vi "Initialise Picture Ring Array.vi"(8 "error in (no error)":errorcluster, 10 "Selection Grid":T1) -> (0 "error out":errorcluster, 1 "Valid":bool, 3 "Grassfire 2D out":refnum<class "Grassfire 2D.lvclass">)   [LabVIEW 2019, in "Grassfire 2D.lvclass"]
uses:
  Grassfire 2D.lvclass
  Shared/Selection--array.ctl
  Shared/Selection--picture ring.ctl
  Node Address--cluster.ctl
  Node Value--cluster.ctl
  Shared/Node Type--enum.ctl
  Grassfire 2D.lvclass/Grassfire 2D.ctl
  Shared/Shared.lvlib
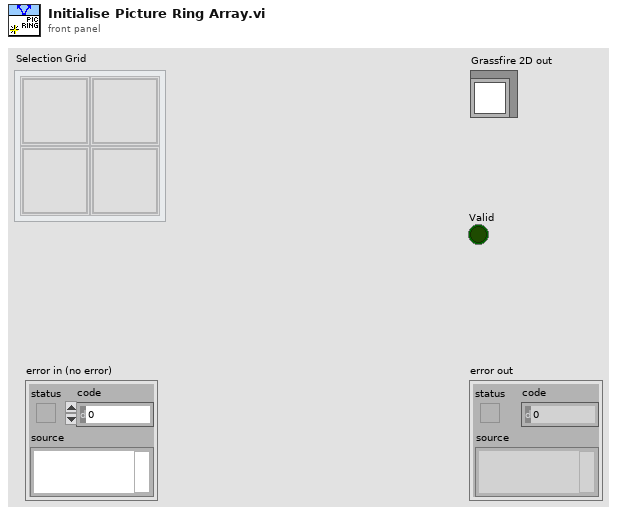
[diagram p1: front panel]
types:
  T1 = typedef "Shared.lvlib/Selection--array.ctl" = cluster{"Grid Value":T2}[][]
  T2 = typedef "Shared.lvlib/Selection--picture ring.ctl" = i64
  T3 = typedef "Grassfire 2D.lvclass/Node Address--cluster.ctl" = cluster{"Row":i32, "Column":i32}
  T4 = typedef "Grassfire 2D.lvclass/Node Value--cluster.ctl" = cluster{"Type":T5, "Distance":i32}
  T5 = typedef "Shared.lvlib/Node Type--enum.ctl" = enum16{"Empty", "Blocked", "Start", "End", "Path"}
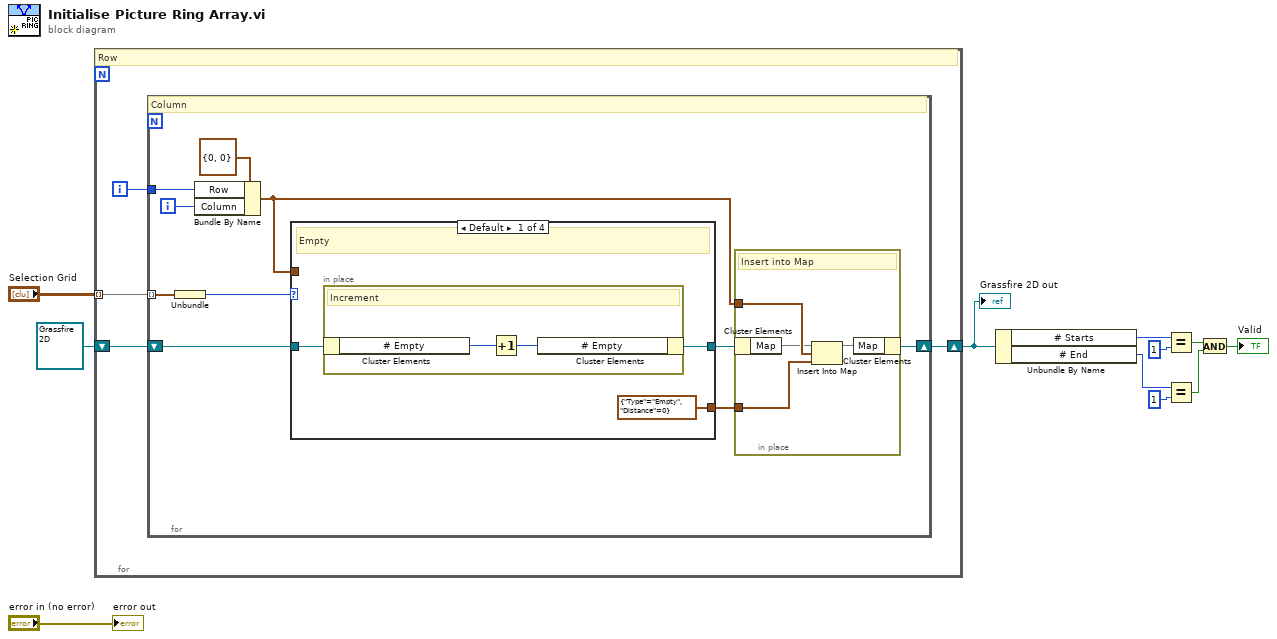
[diagram p0: block diagram]
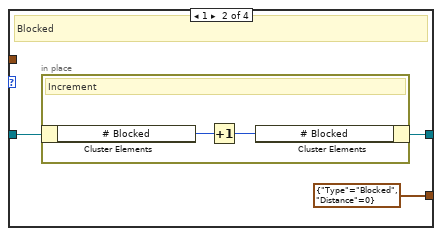
[diagram p2: hidden frame]
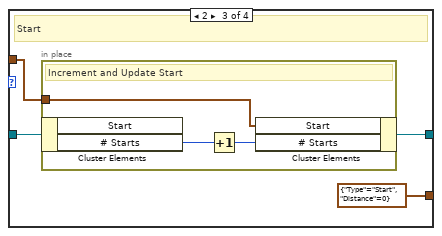
[diagram p3: hidden frame]
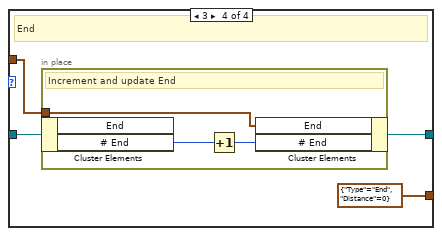
[diagram p4: hidden frame]
diagram:
  n1 = for {
    shift-right: [w13] -> w2
    shift-left: refnum<class "Grassfire 2D.lvclass"> refnum ("Grassfire 2D out") -> [w15]
    tunnel: "Selection Grid" -> [w14] mode=indexing
    i -> [w12]
    # "Row"
    n2 = for {
      shift-right: [w21] -> w13
      shift-left: w15 -> [w23]
      tunnel: w14 -> [w25] mode=indexing
      tunnel: w12 -> [w19]
      i -> [w18]
      # "Column"
      n3 = Unbundle(w25) -> ("Grid Value"=w24:T2)
      n4 = Bundle By Name(cluster=T3 {"Row"=0, "Column"=0} ("Address"), "Row"=w19, "Column"=w18) -> (w16:T3)
      n5 = case shown="Default" w24 {
        tunnel: w23 -> [w32 w37 w43 w50]
        tunnel: [w31 w36 w42 w49] -> w22
        tunnel: [T4 {"Type"=enum."Empty", "Distance"=0} ("Value") T4 {"Type"=enum."Blocked", "Distance"=0} ("Value") T4 {"Type"=enum."Start", "Distance"=0} ("Value") T4 {"Type"=enum."End", "Distance"=0} ("Value")] -> w17
        tunnel: w16 -> [_ _ w40 w48]
        frame Default {
          # "Empty"
          n6 = in-place {
            # "Increment"
            n7 = in-place-cluster #1(w32) -> ("# Empty"=w34:i32)
            n8 = Increment(x=w34) -> (x+1=w33:i32)
            n9 = in-place-cluster #1("# Empty"=w33) -> (w31:refnum<class "Grassfire 2D.lvclass">)
          }
        }
        frame 1 {
          # "Blocked"
          n10 = in-place {
            # "Increment"
            n11 = in-place-cluster #2(w37) -> ("# Blocked"=w39:i32)
            n12 = Increment(x=w39) -> (x+1=w38:i32)
            n13 = in-place-cluster #2("# Blocked"=w38) -> (w36:refnum<class "Grassfire 2D.lvclass">)
          }
        }
        frame 2 {
          # "Start"
          n14 = in-place {
            in-place-border: w40 -> [w44]
            # "Increment and Update Start"
            n15 = in-place-cluster #3(w43) -> ("# Starts"=w46:i32)  [unwired: 1 out]
            n16 = Increment(x=w46) -> (x+1=w45:i32)
            n17 = in-place-cluster #3("Start"=w44, "# Starts"=w45) -> (w42:refnum<class "Grassfire 2D.lvclass">)
          }
        }
        frame 3 {
          # "End"
          n18 = in-place {
            in-place-border: w48 -> [w51]
            # "Increment and update End"
            n19 = in-place-cluster #4(w50) -> ("# End"=w53:i32)  [unwired: 1 out]
            n20 = Increment(x=w53) -> (x+1=w52:i32)
            n21 = in-place-cluster #4("End"=w51, "# End"=w52) -> (w49:refnum<class "Grassfire 2D.lvclass">)
          }
        }
      }
      n22 = in-place {
        in-place-border: w16 -> [w27]
        in-place-border: w17 -> [w28]
        # "Insert into Map"
        n23 = in-place-cluster #5(w22) -> ("Map"=w26:map{T3, T4})
        n24 = Insert Into Map(map in=w26, key=w27, value=w28) -> (map out=w29:map{T3, T4})  [unwired: 2 out]
        n25 = in-place-cluster #5("Map"=w29) -> (w21:refnum<class "Grassfire 2D.lvclass">)
      }
    }
  }
  "Grassfire 2D out" <- w2
  n26 = Unbundle By Name(w2) -> ("# Starts"=w9:i32, "# End"=w10:i32)
  n27 = Equal?(x=w9, y=1) -> (x = y?=w6:bool)
  n28 = Equal?(x=w10, y=1) -> (x = y?=w8:bool)
  n29 = And(x=w6, y=w8) -> (x .and. y?=→"Valid":bool)
  "error out" <- "error in (no error)"
